vi "Read Transaction ID.vi"(11 "IP Data Unit in":refnum<class "IP Data Unit.lvclass">) -> (2 "Transaction ID":u16, 3 "IP Data Unit out":refnum<class "IP Data Unit.lvclass">)   [LabVIEW 2021, in "IP Data Unit.lvclass"]
uses:
  IP Data Unit.lvclass
  IP Data Unit.lvclass/IP Data Unit.ctl
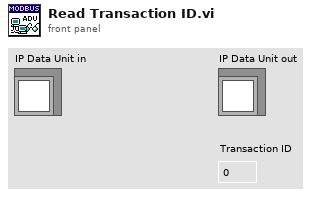
[diagram p1: front panel]
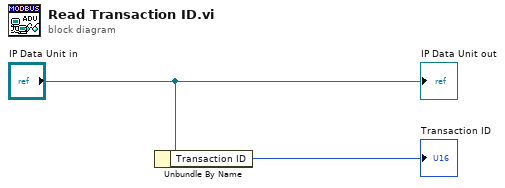
[diagram p0: block diagram]
diagram:
  n1 = Unbundle By Name("IP Data Unit in") -> ("Transaction ID"=→"Transaction ID":u16)
  "IP Data Unit out" <- "IP Data Unit in"
